vi "change path format.vi"(11 "conflicted files list in":string[](array[string])) -> (3 "conflicted files list out":string[](array[string]))   [LabVIEW 2022 SP3]
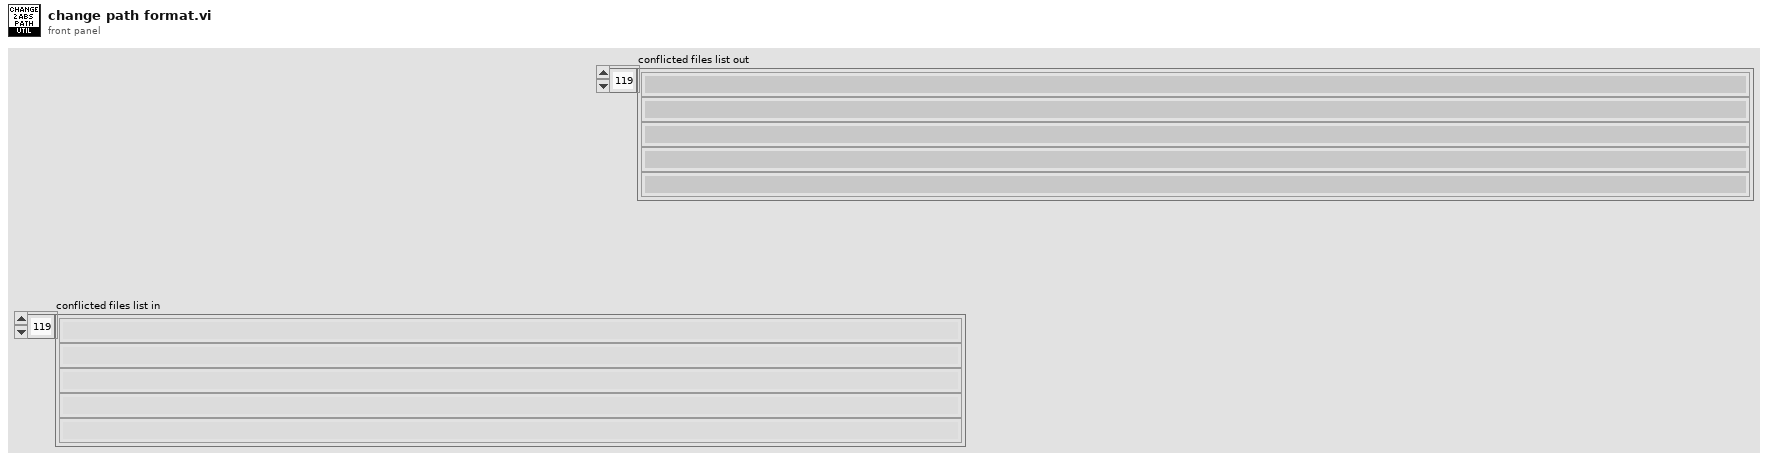
[diagram p1: front panel]
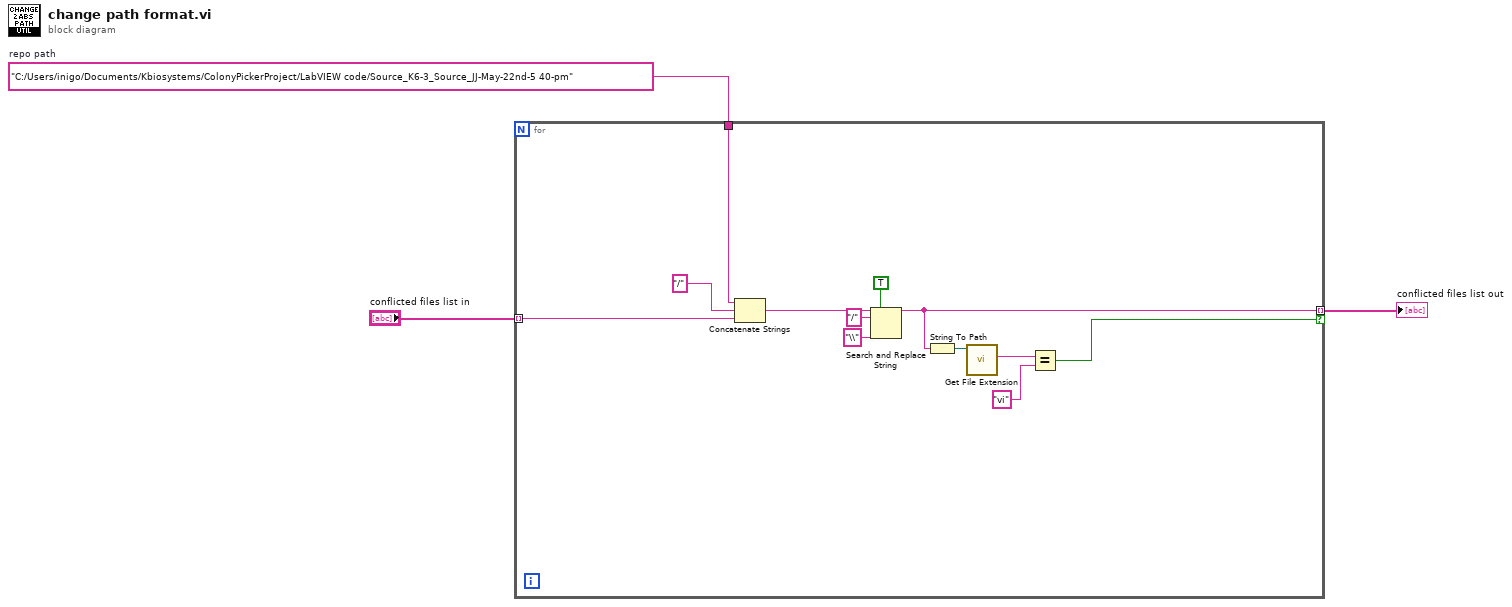
[diagram p0: block diagram]
diagram:
  w2 = "C:/Users/inigo/Documents/Kbiosystems/ColonyPickerProject/LabVIEW code/Source_K6-3_Source_JJ-May-22nd-5 40-pm"  # repo path
  n1 = for {
    tunnel: "conflicted files list in" -> [w15] mode=indexing
    tunnel: w2 -> [w13]
    tunnel: [w7] -> w1 mode=indexing if=w4
    n2 = Concatenate Strings(w13, "/" ("string"), w15) -> (w12:string)
    n3 = Search and Replace String(replace all?=TRUE ("replace all? (F)"), input string=w12, search string="/", replace string="\\" ("replace string (\"\")")) -> (result string=w7:string)  [unwired: 4 in, 3 out]
    n4 = String To Path(string=w7) -> (path=w8:path)
    n5 = call <vilib>:"Get File Extension.vi"("file"=w8) -> ("lowercase file extension"=w6:string)  [unwired: 6 in, 4 out]
    n6 = Equal?(x=w6, y="vi") -> (x = y?=w4:bool)
  }
  "conflicted files list out" <- w1
